vi "Sub_Set_OutputShapePulseDelayWidth.vi"(2 "APERTURE_TIME":dbl=0.0001, 3 "PULSE_WIDTH":dbl=0.001, 4 "error in (no error)":errorcluster, 5 "PULSE_DELAY":dbl=0.0005, 6 "i":i32, 7 "AgB29xxLib.IAgB29xx2":refnum<k7>) -> (0 "error out":errorcluster, 1 "AgB29xxLib.IAgB29xx2 2":refnum<k7>)   [LabVIEW 2009]
panel:
  # "Sub VI: Set Output Wave Shape Pulse Delay Width"
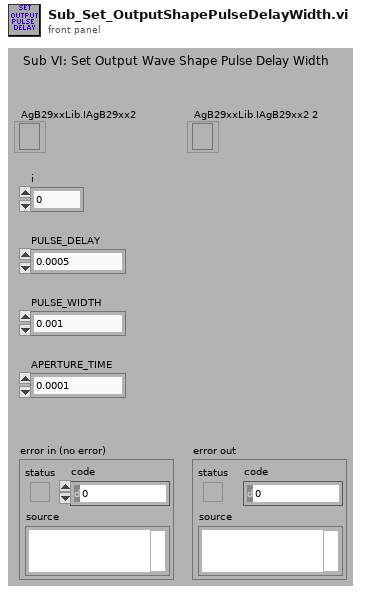
[diagram p1: front panel]
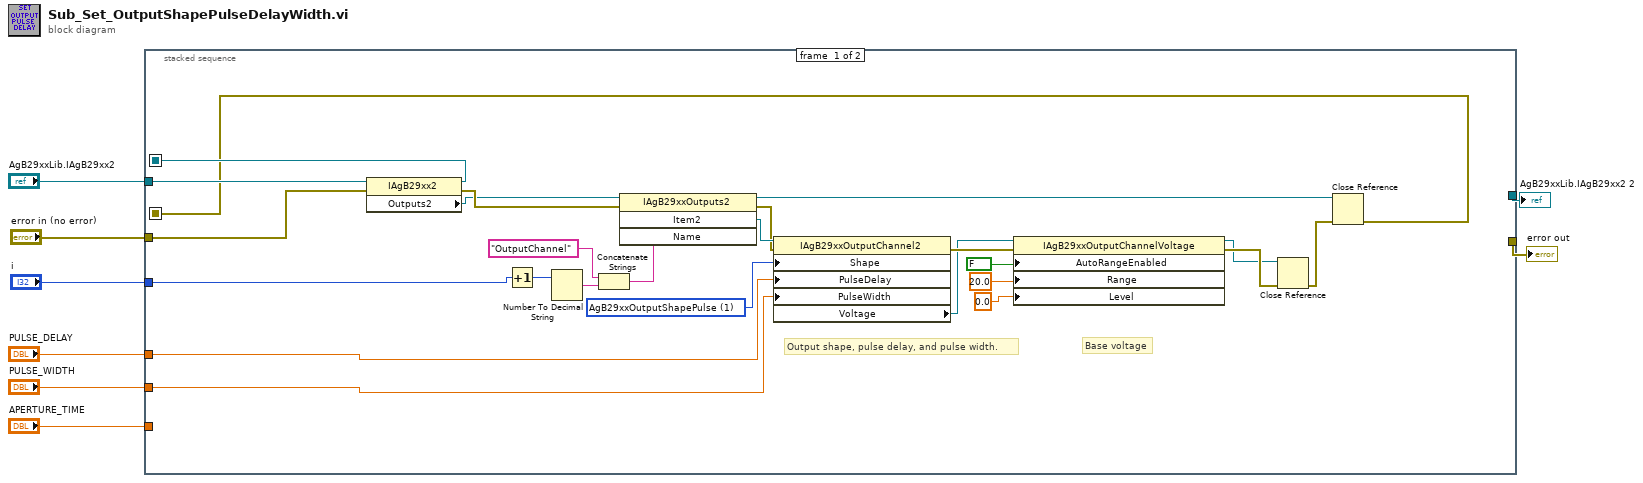
[diagram p0: block diagram]
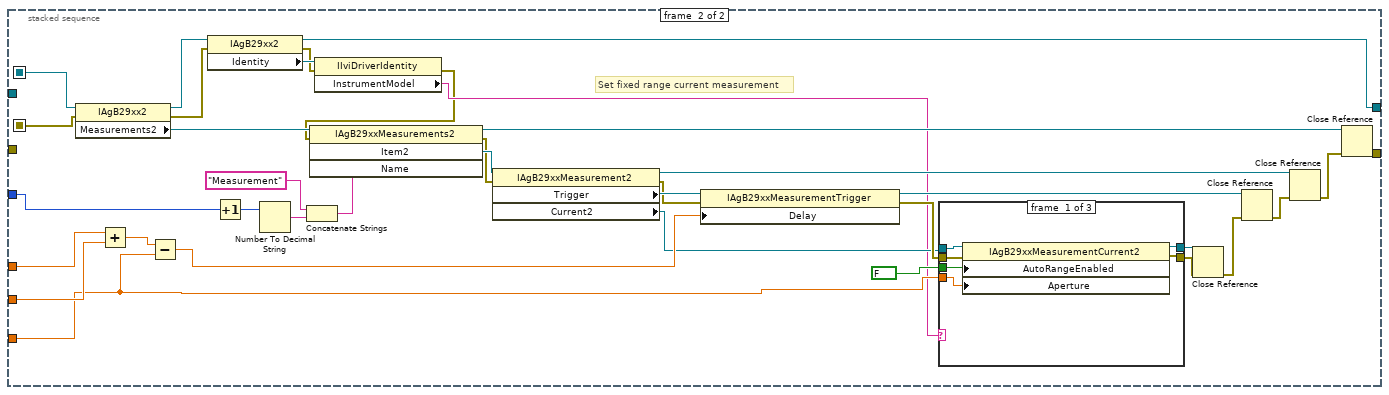
[diagram p2: hidden frame]
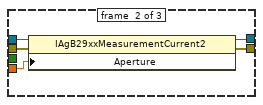
[diagram p3: hidden frame]
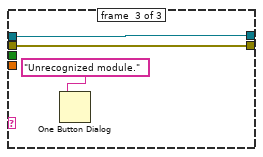
[diagram p4: hidden frame]
diagram:
  n1 = stacked-sequence {
    seq-local: [w30 _] -> [_ w66]
    seq-local: [w29 _] -> [_ w65]
    tunnel: "i" -> [w10 w47]
    tunnel: "PULSE_WIDTH" -> [w33 w68]
    tunnel: "PULSE_DELAY" -> [w32 w69]
    tunnel: "AgB29xxLib.IAgB29xx2" -> [w31 _]
    tunnel: "APERTURE_TIME" -> [_ w41]
    tunnel: [_ w35] -> w3
    tunnel: [_ w67] -> w2
    tunnel: "error in (no error)" -> [w28 _]
    frame #0 {
      w16 = 1 items=["AgB29xxOutputShapeDC", "AgB29xxOutputShapePulse"] ("Shape")
      # "Base voltage"
      # "Output shape, pulse delay, and pulse width."
      n2 = property class="IAgB29xx2"(reference=w31, error in=w28) -> (reference out=w30:refnum<k7>, error out=w27:errorcluster, "Outputs2"=w26:refnum<k7>)
      n3 = Increment(x=w10) -> (x+1=w11:i32)
      n4 = Number To Decimal String(number=w11) -> (decimal integer string=w24:string)  [unwired: 1 in]
      n5 = Concatenate Strings("OutputChannel" ("string"), w24) -> (w22:string)
      n6 = invoke class="IAgB29xxOutputs2" method="Item2"(reference=w26, error in=w27, "Name"=w22) -> (reference out=w17:refnum<k7>, error out=w20:errorcluster, "Item2"=w25:refnum<k7>)  [unwired: 1 in, 1 out]
      n7 = property class="IAgB29xxOutputChannel2"(reference=w25, error in=w20, "Shape"=w16, "PulseDelay"=w32, "PulseWidth"=w33) -> (error out=w21:errorcluster, "Voltage"=w9:refnum<k7>)  [unwired: 1 out]
      n8 = property class="IAgB29xxOutputChannelVoltage"(reference=w9, error in=w21, "AutoRangeEnabled"=FALSE, "Range"=20.0, "Level"=0.0 ("Range")) -> (reference out=w18:refnum<k7>, error out=w19:errorcluster)
      n9 = Close Reference(reference=w18, error in (no error)=w19) -> (error out=w15:errorcluster)
      n10 = Close Reference(reference=w17, error in (no error)=w15) -> (error out=w29:errorcluster)
    }
    frame #1 {
      # "Set fixed range current measurement"
      n11 = property class="IAgB29xx2"(reference=w66, error in=w65) -> (reference out=w40:refnum<k7>, error out=w39:errorcluster, "Measurements2"=w64:refnum<k7>)
      n12 = Add(x=w69, y=w68) -> (x+y=w63:dbl)
      n13 = Subtract(x=w63, y=w41) -> (x-y=w62:dbl)
      n14 = property class="IAgB29xx2"(reference=w40, error in=w39) -> (reference out=w35:refnum<k7>, error out=w37:errorcluster, "Identity"=w38:refnum<k7>)
      n15 = Increment(x=w47) -> (x+1=w60:i32)
      n16 = Number To Decimal String(number=w60) -> (decimal integer string=w59:string)  [unwired: 1 in]
      n17 = Concatenate Strings("Measurement" ("string"), w59) -> (w57:string)
      n18 = property class="IIviDriverIdentity"(reference=w38, error in=w37) -> (error out=w34:errorcluster, "InstrumentModel"=w36:string)  [unwired: 1 out]
      n19 = invoke class="IAgB29xxMeasurements2" method="Item2"(reference=w64, error in=w34, "Name"=w57) -> (reference out=w49:refnum<k7>, error out=w54:errorcluster, "Item2"=w61:refnum<k7>)  [unwired: 1 in, 1 out]
      n20 = property class="IAgB29xxMeasurement2"(reference=w61, error in=w54) -> (reference out=w51:refnum<k7>, error out=w55:errorcluster, "Trigger"=w56:refnum<k7>, "Current2"=w43:refnum<k7>)
      n21 = property class="IAgB29xxMeasurementTrigger"(reference=w56, error in=w55, "Delay"=w62) -> (reference out=w53:refnum<k7>, error out=w44:errorcluster)
      n22 = case shown="\"B2961A\", \"B2962A\"" w36 {
        tunnel: [w75 w80 w82] -> w46
        tunnel: [w74 w79 w81] -> w45
        tunnel: w43 -> [w73 w77 w82]
        tunnel: w44 -> [w72 w78 w81]
        tunnel: w41 -> [w70 w76 _]
        tunnel: FALSE ("AutoRangeEnabled") -> [w71 _ _]
        frame #0 {
          n23 = property class="IAgB29xxMeasurementCurrent2"(reference=w73, error in=w72, "AutoRangeEnabled"=w71, "Aperture"=w70) -> (reference out=w75:refnum<k7>, error out=w74:errorcluster)
        }
        frame #1 {
          n24 = property class="IAgB29xxMeasurementCurrent2"(reference=w77, error in=w78, "Aperture"=w76) -> (reference out=w80:refnum<k7>, error out=w79:errorcluster)
        }
        frame #2 {
          n25 = One Button Dialog(message="Unrecognized module.") -> ()  [unwired: 1 in, 1 out]
        }
      }
      n26 = Close Reference(reference=w46, error in (no error)=w45) -> (error out=w48:errorcluster)
      n27 = Close Reference(reference=w53, error in (no error)=w48) -> (error out=w52:errorcluster)
      n28 = Close Reference(reference=w51, error in (no error)=w52) -> (error out=w50:errorcluster)
      n29 = Close Reference(reference=w49, error in (no error)=w50) -> (error out=w67:errorcluster)
    }
  }
  "error out" <- w2
  "AgB29xxLib.IAgB29xx2 2" <- w3
